vi "filtro Adaptativo LV ECG.vi"() -> ()   [LabVIEW 2014]
doc: "This example demonstrates how to extract fetal electrocardiogram (ECG) signals from maternal abdominal ECG signals. You obtain maternal abdominal ECG signals from obdominal leads. Maternal abdominal ECG signals contain both maternal ECG signals and fetal ECG signals. You can use an adaptive filter to extract fetal ECG signals from maternal abdominal ECG signals. To use an adaptive filter as the solution, you must obtain maternal thorax ECG signals from thorax leads as reference signals."
uses:
  Documents/sd_2015_2/Control 1.ctl
  <vilib>/addons/Adaptive Filters/Create/AFT Create FIR LMS (Real).vi
  <vilib>/addons/Adaptive Filters/Processing/AFT Filter Signal and Update Coefficients (Real, Array).vi
  <vilib>/addons/Adaptive Filters/NI_AdaptiveFilter.lvlib
  <vilib>/Analysis/NI_AALBase.lvlib
panel:
  in  "Step Size":T1=0.45 min=0.0 step=0.01 format="%#_9f"
  in  "Filter Length":i32=40 min=2
  out "Fetal ECG":dbl[](graph)
  out "Waveform Graph 3":dbl[](graph)
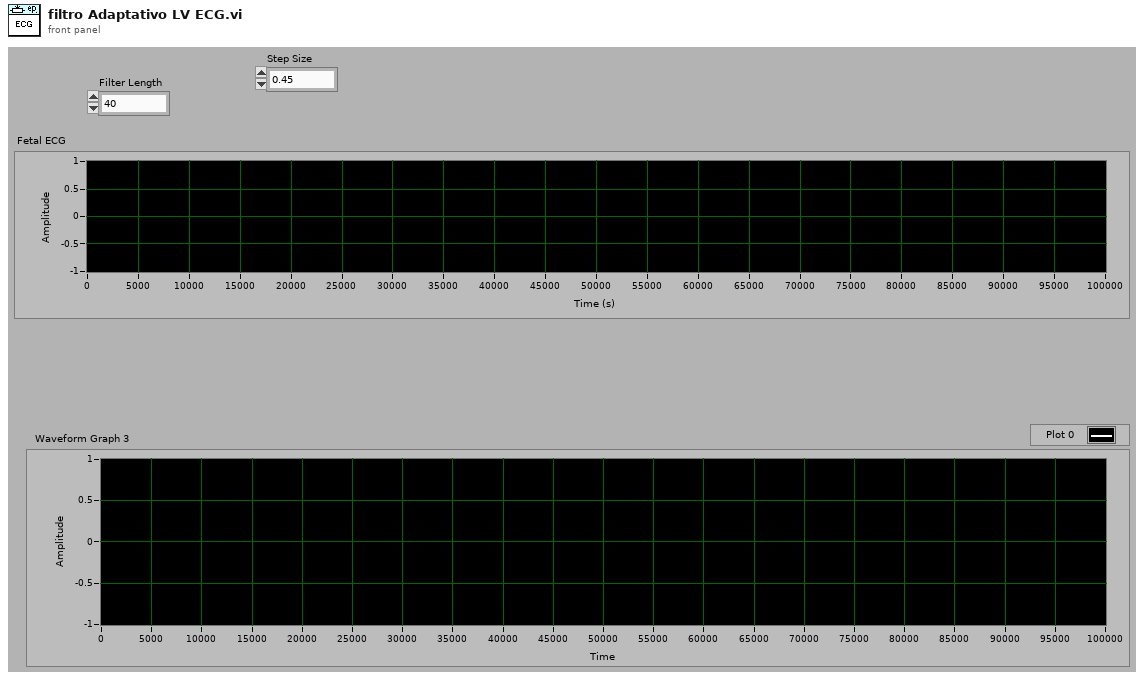
[diagram p1: front panel]
types:
  T1 = typedef "Control 1.ctl" = dbl
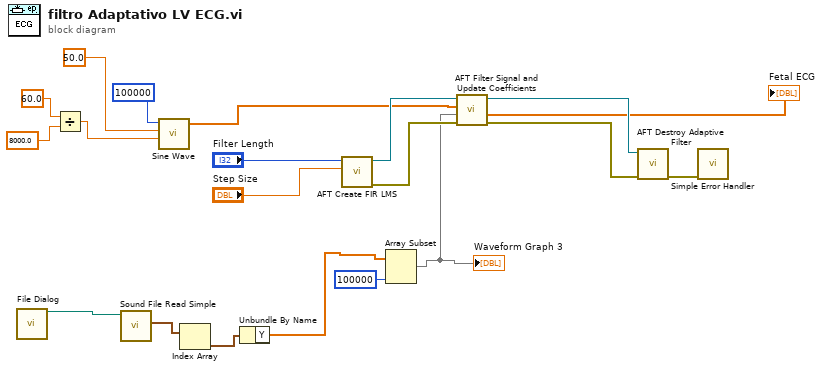
[diagram p0: block diagram]
diagram:
  n1 = call "File Dialog"() -> ("selected path"=w4:path)  [unwired: 12 in, 3 out]
  n2 = Divide(x=60.0, y=8000.0) -> (x/y=w12:dbl)
  n3 = call <vilib>:"Sound File Read Simple.vi"("path"=w4) -> ("data"=w3:waveform(dbl)[])  [unwired: 7 in, 3 out]
  n4 = call <vilib>:"Sine Wave.vi"("samples"=100000, "amplitude"=50.0, "frequency"=w12) -> ("sine wave"=w7:dbl[])  [unwired: 2 in, 2 out]
  n5 = Index Array(array=w3) -> (element=w2:waveform(dbl))  [unwired: 1 in]
  n6 = Unbundle By Name(w2) -> ("Y"=w1:dbl[])
  n7 = call-poly <vilib>:"AFT Create FIR LMS.vi"("step size"="Step Size", "filter length"="Filter Length") -> ("error out"=w15:errorcluster, "adaptive filter out"=w16:refnum<k20>)  [unwired: 2 in, 6 out]
  n8 = Array Subset(array=w1, length=100000) -> (w8:dbl[])  [unwired: 1 in]
  "Waveform Graph 3" <- w8
  n9 = call-poly <vilib>:"AFT Filter Signal and Update Coefficients.vi"("error in (no error)"=w15, "d(n)"=w8, "x(n)"=w7, "adaptive filter in"=w16) -> ("error out"=w19:errorcluster, "e(n)"=→"Fetal ECG":dbl[], "adaptive filter out"=w20:refnum<k20>)  [unwired: 2 in, 3 out]
  n10 = call <vilib>:"AFT Destroy Adaptive Filter.vi"("error in (no error)"=w19, "adaptive filter in"=w20) -> ("error out"=w14:errorcluster)  [unwired: 9 out]
  n11 = call <vilib>:"Simple Error Handler.vi"("error in (no error)"=w14) -> ()  [unwired: 1 in, 8 out]
